vi "BMU诊断标定.vi"(8 "CAN端口":u16(ring), 9 "设备索引号":u16(ring), 10 "CAN卡类型":u32(ring)=21) -> ()   [LabVIEW 2013] (continued)
                n969 = Index Array(array=w1309, index=5 ("索引")) -> (element=w1308:bool)
                n970 = Not(x=w1317) -> (.not. x?=w1316:bool)
              }
              frame "温度起始值" {
                w1353 = 2
                w1355 = FALSE
                n971 = property on="电池实际容量(A)" class="DigNum (严格)"("Disabled"=w1353) -> ()  [unwired: 2 in, 2 out]
                n972 = property on="使用者" class="DigNum (严格)"("Disabled"=w1353) -> ()  [unwired: 2 in, 2 out]
                n973 = property on="SOH(%)" class="DigNum (严格)"("Disabled"=w1353) -> ()  [unwired: 2 in, 2 out]
                n974 = property on="电池额定容量(A)" class="DigNum (严格)"("Disabled"=w1353) -> ()  [unwired: 2 in, 2 out]
                n975 = property on="SOC(%)" class="DigNum (严格)"("Disabled"=w1353) -> ()  [unwired: 2 in, 2 out]
                n976 = local read "从板个数"() -> (w1351:dbl)
                n977 = property on="系统时钟" class="Str"("Disabled"=w1353) -> ()  [unwired: 2 in, 2 out]
                n978 = property on="配置文件版本" class="Str"("Disabled"=w1353) -> ()  [unwired: 2 in, 2 out]
                n979 = property on="车架(牌)号" class="Str"("Disabled"=w1353) -> ()  [unwired: 2 in, 2 out]
                n980 = property on="产品编号" class="Str"("Disabled"=w1353) -> ()  [unwired: 2 in, 2 out]
                n981 = control-ref of="项目信息"() -> (w1352:refnum<vi>)
                n982 = stacked-sequence {
                  tunnel: w1352 -> [w1364 w1367 w1380]
                  tunnel: w1351 -> [w1357 w1366 w1379]
                  frame #0 {
                    n983 = Multiply(x=w1357, y=3.0) -> (x*y=w1359:dbl)
                    n984 = Compound Arithmetic op=ADD(23.0 ("值"), w1359) -> (w1361:dbl)
                    n985 = Bundle(w1361, 0) -> (w1363:cluster{dbl, i32})  [unwired: 1 out]
                    n986 = property class="Tbl (严格)"(reference=w1364, "Index Values"=w1363) -> ()  [unwired: 1 in, 2 out]
                  }
                  frame #1 {
                    n987 = for {
                      N: 10 -> [_]
                      tunnel: w1367 -> [w1377]
                      tunnel: w1366 -> [w1372]
                      i -> [w1371]
                      n988 = Multiply(x=4.0, y=w1372) -> (x*y=w1369:dbl)
                      n989 = Compound Arithmetic op=ADD(24.0 ("值"), w1369, w1371) -> (w1374:dbl)
                      n990 = Bundle(w1374, 0) -> (w1376:cluster{dbl, i32})  [unwired: 1 out]
                      n991 = property class="Tbl (严格)"(reference=w1377, "Active Cell"=w1376, "Cell BG Color"=u32 16448250) -> ()  [unwired: 1 in, 2 out]
                    }
                  }
                  frame #2 {
                    n992 = Increment(x=w1379) -> (x+1=w1378:dbl)
                    n993 = for {
                      N: w1378 -> [_]
                      tunnel: w1380 -> [w1390]
                      tunnel: w1379 -> [w1385]
                      i -> [w1384]
                      n994 = Multiply(x=3.0, y=w1385) -> (x*y=w1382:dbl)
                      n995 = Compound Arithmetic op=ADD(23.0 ("值"), w1382, w1384) -> (w1387:dbl)
                      n996 = Bundle(w1387, 0) -> (w1389:cluster{dbl, i32})  [unwired: 1 out]
                      n997 = property class="Tbl (严格)"(reference=w1390, "Active Cell"=w1389, "Cell BG Color"=u32 6618880) -> ()  [unwired: 1 in, 2 out]
                    }
                  }
                }
                n998 = Select(t=0, s=w1342, f=1) -> (s? t:f=w1341:i32)
                n999 = property on="从板个数" class="DigNum (严格)"("NumText.BGColor"=u32 13816530) -> ()  [unwired: 2 in, 2 out]
                n1000 = property on="项目信息" class="Tbl (严格)"("Disabled"=w1341) -> ()  [unwired: 2 in, 2 out]
                n1001 = global read "功能码全局.vi" "主板项目信息5"() -> (w1349:bool[])
                n1002 = global read "功能码全局.vi" "主板项目信息6"() -> (w1347:bool[])
                n1003 = Index Array(array=w1349, index=5 ("索引")) -> (element=w1346:bool)
                n1004 = Index Array(array=w1347, index=6 ("索引")) -> (element=w1345:bool)
                n1005 = Not(x=w1355) -> (.not. x?=w1354:bool)
              }
              frame "保险位置" {
                w1403 = 2
                w1405 = FALSE
                n1006 = property on="电池实际容量(A)" class="DigNum (严格)"("Disabled"=w1403) -> ()  [unwired: 2 in, 2 out]
                n1007 = property on="使用者" class="DigNum (严格)"("Disabled"=w1403) -> ()  [unwired: 2 in, 2 out]
                n1008 = property on="SOH(%)" class="DigNum (严格)"("Disabled"=w1403) -> ()  [unwired: 2 in, 2 out]
                n1009 = property on="电池额定容量(A)" class="DigNum (严格)"("Disabled"=w1403) -> ()  [unwired: 2 in, 2 out]
                n1010 = property on="SOC(%)" class="DigNum (严格)"("Disabled"=w1403) -> ()  [unwired: 2 in, 2 out]
                n1011 = local read "从板个数"() -> (w1401:dbl)
                n1012 = property on="系统时钟" class="Str"("Disabled"=w1403) -> ()  [unwired: 2 in, 2 out]
                n1013 = property on="配置文件版本" class="Str"("Disabled"=w1403) -> ()  [unwired: 2 in, 2 out]
                n1014 = property on="车架(牌)号" class="Str"("Disabled"=w1403) -> ()  [unwired: 2 in, 2 out]
                n1015 = property on="产品编号" class="Str"("Disabled"=w1403) -> ()  [unwired: 2 in, 2 out]
                n1016 = control-ref of="项目信息"() -> (w1402:refnum<vi>)
                n1017 = stacked-sequence {
                  tunnel: w1402 -> [w1414 w1417]
                  tunnel: w1401 -> [w1407 w1416]
                  frame #0 {
                    n1018 = Multiply(x=w1407, y=4.0) -> (x*y=w1409:dbl)
                    n1019 = Compound Arithmetic op=ADD(24.0 ("值"), w1409) -> (w1411:dbl)
                    n1020 = Bundle(w1411, 0) -> (w1413:cluster{dbl, i32})  [unwired: 1 out]
                    n1021 = property class="Tbl (严格)"(reference=w1414, "Index Values"=w1413) -> ()  [unwired: 1 in, 2 out]
                  }
                  frame #1 {
                    n1022 = for {
                      N: 20 -> [_]
                      tunnel: w1417 -> [w1427]
                      tunnel: w1416 -> [w1422]
                      i -> [w1421]
                      n1023 = Multiply(x=4.0, y=w1422) -> (x*y=w1419:dbl)
                      n1024 = Compound Arithmetic op=ADD(24.0 ("值"), w1419, w1421) -> (w1424:dbl)
                      n1025 = Bundle(w1424, 0) -> (w1426:cluster{dbl, i32})  [unwired: 1 out]
                      n1026 = property class="Tbl (严格)"(reference=w1427, "Active Cell"=w1426, "Cell BG Color"=u32 6618880) -> ()  [unwired: 1 in, 2 out]
                    }
                  }
                }
                n1027 = property on="从板个数" class="DigNum (严格)"("NumText.BGColor"=u32 13816530) -> ()  [unwired: 2 in, 2 out]
                n1028 = Select(t=0, s=w1394, f=1) -> (s? t:f=w1392:i32)
                n1029 = global read "功能码全局.vi" "主板项目信息4"() -> (w1399:bool[])
                n1030 = property on="项目信息" class="Tbl (严格)"("Disabled"=w1392) -> ()  [unwired: 2 in, 2 out]
                n1031 = Index Array(array=w1399, index #1=5 ("索引"), index #2=6 ("索引")) -> (element #1=w1397:bool, element #2=w1396:bool)
                n1032 = Not(x=w1405) -> (.not. x?=w1404:bool)
              }
              frame "SOC" {
                w1438 = 2
                w1440 = FALSE
                n1033 = property on="电池实际容量(A)" class="DigNum (严格)"("Disabled"=w1438) -> ()  [unwired: 2 in, 2 out]
                n1034 = property on="使用者" class="DigNum (严格)"("Disabled"=w1438) -> ()  [unwired: 2 in, 2 out]
                n1035 = property on="SOH(%)" class="DigNum (严格)"("Disabled"=w1438) -> ()  [unwired: 2 in, 2 out]
                n1036 = property on="电池额定容量(A)" class="DigNum (严格)"("Disabled"=w1438) -> ()  [unwired: 2 in, 2 out]
                n1037 = property on="从板个数" class="DigNum (严格)"("NumText.BGColor"=u32 13816530) -> ()  [unwired: 2 in, 2 out]
                n1038 = property on="系统时钟" class="Str"("Disabled"=w1438) -> ()  [unwired: 2 in, 2 out]
                n1039 = property on="配置文件版本" class="Str"("Disabled"=w1438) -> ()  [unwired: 2 in, 2 out]
                n1040 = property on="车架(牌)号" class="Str"("Disabled"=w1438) -> ()  [unwired: 2 in, 2 out]
                n1041 = property on="项目信息" class="Tbl (严格)"("Disabled"=w1438) -> ()  [unwired: 2 in, 2 out]
                n1042 = property on="产品编号" class="Str"("Disabled"=w1438) -> ()  [unwired: 2 in, 2 out]
                n1043 = Select(t=0, s=w1430, f=0) -> (s? t:f=w1429:i32)
                n1044 = property on="SOC(%)" class="DigNum (严格)"("Disabled"=w1429) -> ()  [unwired: 2 in, 2 out]
                n1045 = property on="项目信息2" class="Clust (严格)"("DisabledEnum"=w1429) -> ()  [unwired: 2 in, 2 out]
                n1046 = global read "功能码全局.vi" "主板项目信息7"() -> (w1436:bool[])
                n1047 = Index Array(array=w1436, index #1=2 ("索引"), index #2=5 ("索引")) -> (element #1=w1434:bool, element #2=w1433:bool)
                n1048 = Not(x=w1440) -> (.not. x?=w1439:bool)
              }
              frame "电池额定实际容量" {
                w1452 = 2
                w1454 = FALSE
                n1049 = property on="使用者" class="DigNum (严格)"("Disabled"=w1452) -> ()  [unwired: 2 in, 2 out]
                n1050 = property on="SOH(%)" class="DigNum (严格)"("Disabled"=w1452) -> ()  [unwired: 2 in, 2 out]
                n1051 = property on="SOC(%)" class="DigNum (严格)"("Disabled"=w1452) -> ()  [unwired: 2 in, 2 out]
                n1052 = property on="从板个数" class="DigNum (严格)"("NumText.BGColor"=u32 13816530) -> ()  [unwired: 2 in, 2 out]
                n1053 = property on="系统时钟" class="Str"("Disabled"=w1452) -> ()  [unwired: 2 in, 2 out]
                n1054 = property on="配置文件版本" class="Str"("Disabled"=w1452) -> ()  [unwired: 2 in, 2 out]
                n1055 = property on="车架(牌)号" class="Str"("Disabled"=w1452) -> ()  [unwired: 2 in, 2 out]
                n1056 = property on="项目信息" class="Tbl (严格)"("Disabled"=w1452) -> ()  [unwired: 2 in, 2 out]
                n1057 = property on="产品编号" class="Str"("Disabled"=w1452) -> ()  [unwired: 2 in, 2 out]
                n1058 = Select(t=0, s=w1444, f=1) -> (s? t:f=w1443:i32)
                n1059 = property on="电池实际容量(A)" class="DigNum (严格)"("Disabled"=w1443) -> ()  [unwired: 2 in, 2 out]
                n1060 = property on="电池额定容量(A)" class="DigNum (严格)"("Disabled"=w1443) -> ()  [unwired: 2 in, 2 out]
                n1061 = property on="项目信息2" class="Clust (严格)"("DisabledEnum"=w1443) -> ()  [unwired: 2 in, 2 out]
                n1062 = global read "功能码全局.vi" "主板项目信息7"() -> (w1450:bool[])
                n1063 = Index Array(array=w1450, index #1=3 ("索引"), index #2=6 ("索引")) -> (element #1=w1448:bool, element #2=w1447:bool)
                n1064 = Not(x=w1454) -> (.not. x?=w1453:bool)
              }
              frame "配置文件版本" {
                w1467 = 2
                w1469 = FALSE
                n1065 = property on="使用者" class="DigNum (严格)"("Disabled"=w1467) -> ()  [unwired: 2 in, 2 out]
                n1066 = property on="SOH(%)" class="DigNum (严格)"("Disabled"=w1467) -> ()  [unwired: 2 in, 2 out]
                n1067 = property on="SOC(%)" class="DigNum (严格)"("Disabled"=w1467) -> ()  [unwired: 2 in, 2 out]
                n1068 = property on="电池实际容量(A)" class="DigNum (严格)"("Disabled"=w1467) -> ()  [unwired: 2 in, 2 out]
                n1069 = property on="从板个数" class="DigNum (严格)"("NumText.BGColor"=u32 13816530) -> ()  [unwired: 2 in, 2 out]
                n1070 = property on="电池额定容量(A)" class="DigNum (严格)"("Disabled"=w1467) -> ()  [unwired: 2 in, 2 out]
                n1071 = property on="系统时钟" class="Str"("Disabled"=w1467) -> ()  [unwired: 2 in, 2 out]
                n1072 = property on="车架(牌)号" class="Str"("Disabled"=w1467) -> ()  [unwired: 2 in, 2 out]
                n1073 = property on="项目信息" class="Tbl (严格)"("Disabled"=w1467) -> ()  [unwired: 2 in, 2 out]
                n1074 = property on="产品编号" class="Str"("Disabled"=w1467) -> ()  [unwired: 2 in, 2 out]
                n1075 = Select(t=0, s=w1458, f=1) -> (s? t:f=w1457:i32)
                n1076 = property on="项目信息2" class="Clust (严格)"("DisabledEnum"=w1457) -> ()  [unwired: 2 in, 2 out]
                n1077 = property on="配置文件版本" class="Str"("Disabled"=w1457) -> ()  [unwired: 2 in, 2 out]
                n1078 = global read "功能码全局.vi" "主板项目信息5"() -> (w1465:bool[])
                n1079 = global read "功能码全局.vi" "主板项目信息6"() -> (w1464:bool[])
                n1080 = Index Array(array=w1465, index=6 ("索引")) -> (element=w1462:bool)
                n1081 = Index Array(array=w1464, index=7 ("索引")) -> (element=w1461:bool)
                n1082 = Not(x=w1469) -> (.not. x?=w1468:bool)
              }
              frame "参数修改记录" {
                w1482 = 2
                w1484 = FALSE
                n1083 = property on="SOH(%)" class="DigNum (严格)"("Disabled"=w1482) -> ()  [unwired: 2 in, 2 out]
                n1084 = property on="SOC(%)" class="DigNum (严格)"("Disabled"=w1482) -> ()  [unwired: 2 in, 2 out]
                n1085 = property on="电池实际容量(A)" class="DigNum (严格)"("Disabled"=w1482) -> ()  [unwired: 2 in, 2 out]
                n1086 = property on="电池额定容量(A)" class="DigNum (严格)"("Disabled"=w1482) -> ()  [unwired: 2 in, 2 out]
                n1087 = property on="从板个数" class="DigNum (严格)"("NumText.BGColor"=u32 13816530) -> ()  [unwired: 2 in, 2 out]
                n1088 = property on="系统时钟" class="Str"("Disabled"=w1482) -> ()  [unwired: 2 in, 2 out]
                n1089 = property on="车架(牌)号" class="Str"("Disabled"=w1482) -> ()  [unwired: 2 in, 2 out]
                n1090 = property on="配置文件版本" class="Str"("Disabled"=w1482) -> ()  [unwired: 2 in, 2 out]
                n1091 = property on="项目信息" class="Tbl (严格)"("Disabled"=w1482) -> ()  [unwired: 2 in, 2 out]
                n1092 = property on="产品编号" class="Str"("Disabled"=w1482) -> ()  [unwired: 2 in, 2 out]
                n1093 = Select(t=0, s=w1473, f=1) -> (s? t:f=w1472:i32)
                n1094 = property on="使用者" class="DigNum (严格)"("Disabled"=w1472) -> ()  [unwired: 2 in, 2 out]
                n1095 = property on="项目信息2" class="Clust (严格)"("DisabledEnum"=w1472) -> ()  [unwired: 2 in, 2 out]
                n1096 = global read "功能码全局.vi" "主板项目信息7"() -> (w1479:bool[])
                n1097 = global read "功能码全局.vi" "主板项目信息5"() -> (w1480:bool[])
                n1098 = Index Array(array=w1479, index=0 ("索引")) -> (element=w1477:bool)
                n1099 = Index Array(array=w1480, index=7 ("索引")) -> (element=w1476:bool)
                n1100 = Not(x=w1484) -> (.not. x?=w1483:bool)
              }
              frame "车牌号" {
                w1497 = 2
                w1499 = FALSE
                n1101 = property on="SOH(%)" class="DigNum (严格)"("Disabled"=w1497) -> ()  [unwired: 2 in, 2 out]
                n1102 = property on="使用者" class="DigNum (严格)"("Disabled"=w1497) -> ()  [unwired: 2 in, 2 out]
                n1103 = property on="SOC(%)" class="DigNum (严格)"("Disabled"=w1497) -> ()  [unwired: 2 in, 2 out]
                n1104 = property on="电池实际容量(A)" class="DigNum (严格)"("Disabled"=w1497) -> ()  [unwired: 2 in, 2 out]
                n1105 = property on="电池额定容量(A)" class="DigNum (严格)"("Disabled"=w1497) -> ()  [unwired: 2 in, 2 out]
                n1106 = property on="从板个数" class="DigNum (严格)"("NumText.BGColor"=u32 13816530) -> ()  [unwired: 2 in, 2 out]
                n1107 = property on="系统时钟" class="Str"("Disabled"=w1497) -> ()  [unwired: 2 in, 2 out]
                n1108 = property on="配置文件版本" class="Str"("Disabled"=w1497) -> ()  [unwired: 2 in, 2 out]
                n1109 = property on="项目信息" class="Tbl (严格)"("Disabled"=w1497) -> ()  [unwired: 2 in, 2 out]
                n1110 = property on="产品编号" class="Str"("Disabled"=w1497) -> ()  [unwired: 2 in, 2 out]
                n1111 = Select(t=0, s=w1488, f=1) -> (s? t:f=w1487:i32)
                n1112 = property on="车架(牌)号" class="Str"("Disabled"=w1487) -> ()  [unwired: 2 in, 2 out]
                n1113 = property on="项目信息2" class="Clust (严格)"("DisabledEnum"=w1487) -> ()  [unwired: 2 in, 2 out]
                n1114 = global read "功能码全局.vi" "主板项目信息7"() -> (w1494:bool[])
                n1115 = global read "功能码全局.vi" "主板项目信息6"() -> (w1495:bool[])
                n1116 = Index Array(array=w1494, index=1 ("索引")) -> (element=w1492:bool)
                n1117 = Index Array(array=w1495, index=0 ("索引")) -> (element=w1491:bool)
                n1118 = Not(x=w1499) -> (.not. x?=w1498:bool)
              }
              frame "SOH" {
                w1511 = 2
                w1513 = FALSE
                n1119 = property on="使用者" class="DigNum (严格)"("Disabled"=w1511) -> ()  [unwired: 2 in, 2 out]
                n1120 = property on="SOC(%)" class="DigNum (严格)"("Disabled"=w1511) -> ()  [unwired: 2 in, 2 out]
                n1121 = property on="电池实际容量(A)" class="DigNum (严格)"("Disabled"=w1511) -> ()  [unwired: 2 in, 2 out]
                n1122 = property on="电池额定容量(A)" class="DigNum (严格)"("Disabled"=w1511) -> ()  [unwired: 2 in, 2 out]
                n1123 = property on="从板个数" class="DigNum (严格)"("NumText.BGColor"=u32 13816530) -> ()  [unwired: 2 in, 2 out]
                n1124 = property on="系统时钟" class="Str"("Disabled"=w1511) -> ()  [unwired: 2 in, 2 out]
                n1125 = property on="配置文件版本" class="Str"("Disabled"=w1511) -> ()  [unwired: 2 in, 2 out]
                n1126 = property on="项目信息" class="Tbl (严格)"("Disabled"=w1511) -> ()  [unwired: 2 in, 2 out]
                n1127 = property on="产品编号" class="Str"("Disabled"=w1511) -> ()  [unwired: 2 in, 2 out]
                n1128 = property on="车架(牌)号" class="Str"("Disabled"=w1511) -> ()  [unwired: 2 in, 2 out]
                n1129 = Select(t=0, s=w1503, f=1) -> (s? t:f=w1502:i32)
                n1130 = property on="项目信息2" class="Clust (严格)"("DisabledEnum"=w1502) -> ()  [unwired: 2 in, 2 out]
                n1131 = property on="SOH(%)" class="DigNum (严格)"("Disabled"=w1502) -> ()  [unwired: 2 in, 2 out]
                n1132 = global read "功能码全局.vi" "主板项目信息7"() -> (w1510:bool[])
                n1133 = Index Array(array=w1510, index #1=4 ("索引"), index #2=7 ("索引")) -> (element #1=w1507:bool, element #2=w1506:bool)
                n1134 = Not(x=w1513) -> (.not. x?=w1512:bool)
              }
              frame "SOC过低(2)", "SOC过高(2)", "SOH过低(2)", "充电电流过高(2)", "单体电压过低(2)", "单体电压过高(2)", "单组电压不均衡(2)", "单组温度不均衡(2)", "二级故障阀值", "放电电流过高(2)", "极柱温度过高(2)", "内阻过大(2)", "温度过低(2)", "温度过高(2)", "整组电压不均衡(2)", "整组温度不均衡(2)", "总电压过低(2)", "总电压过高(2)" {
                w1525 = FALSE
                n1135 = property on="从板个数" class="DigNum (严格)"("NumText.BGColor"=u32 13816530) -> ()  [unwired: 2 in, 2 out]
                n1136 = Select(t=0, s=w1517, f=1) -> (s? t:f=w1516:i32)
                n1137 = property on="一级故障 2" class="Clust (严格)"("DisabledEnum"=w1516) -> ()  [unwired: 2 in, 2 out]
                n1138 = global read "功能码全局.vi" "主板故障阀值9"() -> (w1523:bool[])
                n1139 = Index Array(array=w1523, index #1=3 ("索引"), index #2=6 ("索引")) -> (element #1=w1521:bool, element #2=w1520:bool)
                n1140 = Not(x=w1525) -> (.not. x?=w1526:bool)
              }
              frame "SOC过低(3)", "SOC过高(3)", "SOH过低(3)", "充电电流过高(3)", "单体电压过低(3)", "单体电压过高(3)", "单组电压不均衡(3)", "单组温度不均衡(3)", "放电电流过高(3)", "极柱温度过高(3)", "内阻过大(3)", "三级故障阀值", "温度过低(3)", "温度过高(3)", "整组电压不均衡(3)", "整组温度不均衡(3)", "总电压过低(3)", "总电压过高(3)" {
                w1539 = FALSE
                n1141 = property on="从板个数" class="DigNum (严格)"("NumText.BGColor"=u32 13816530) -> ()  [unwired: 2 in, 2 out]
                n1142 = Select(t=0, s=w1530, f=1) -> (s? t:f=w1529:i32)
                n1143 = property on="一级故障 3" class="Clust (严格)"("DisabledEnum"=w1529) -> ()  [unwired: 2 in, 2 out]
                n1144 = global read "功能码全局.vi" "主板故障阀值9"() -> (w1536:bool[])
                n1145 = Index Array(array=w1536, index #1=4 ("索引"), index #2=7 ("索引")) -> (element #1=w1534:bool, element #2=w1533:bool)
                n1146 = Not(x=w1539) -> (.not. x?=w1538:bool)
              }
              frame "SOC过低", "SOC过高", "SOH过低", "充电电流过高", "单体电压过低", "单体电压过高", "单组电压不均衡", "单组温度不均衡", "放电电流过高", "极柱温度过高", "内阻过大", "温度过低", "温度过高", "一级故障阀值", "整组电压不均衡", "整组温度不均衡", "总电压过低", "总电压过高" {
                w1552 = FALSE
                n1147 = Select(t=0, s=w1543, f=1) -> (s? t:f=w1542:i32)
                n1148 = property on="从板个数" class="DigNum (严格)"("NumText.BGColor"=u32 13816530) -> ()  [unwired: 2 in, 2 out]
                n1149 = property on="一级故障" class="Clust (严格)"("DisabledEnum"=w1542) -> ()  [unwired: 2 in, 2 out]
                n1150 = global read "功能码全局.vi" "主板故障阀值9"() -> (w1549:bool[])
                n1151 = Index Array(array=w1549, index #1=2 ("索引"), index #2=5 ("索引")) -> (element #1=w1547:bool, element #2=w1546:bool)
                n1152 = Not(x=w1552) -> (.not. x?=w1551:bool)
              }
              frame "充电控制参数", "电流步长", "最大允许充电电流", "最大允许充电温度", "最大允许单体电压", "最大允许总电压", "最小允许充电电流", "最小允许充电温度", "最小允许单体电压" {
                w1555 = 2
                w1566 = FALSE
                n1153 = property on="从板个数" class="DigNum (严格)"("NumText.BGColor"=u32 13816530) -> ()  [unwired: 2 in, 2 out]
                n1154 = property on="风机开启温度" class="DigNum (严格)"("Disabled"=w1555) -> ()  [unwired: 2 in, 2 out]
                n1155 = property on="风机关闭温度" class="DigNum (严格)"("Disabled"=w1555) -> ()  [unwired: 2 in, 2 out]
                n1156 = property on="加热开启温度" class="DigNum (严格)"("Disabled"=w1555) -> ()  [unwired: 2 in, 2 out]
                n1157 = property on="加热关闭温度" class="DigNum (严格)"("Disabled"=w1555) -> ()  [unwired: 2 in, 2 out]
                n1158 = property on="风机开启温差" class="DigNum (严格)"("Disabled"=w1555) -> ()  [unwired: 2 in, 2 out]
                n1159 = property on="风机关闭温差" class="DigNum (严格)"("Disabled"=w1555) -> ()  [unwired: 2 in, 2 out]
                n1160 = property on="加热控制参数" class="Clust (严格)"("DisabledEnum"=w1555) -> ()  [unwired: 2 in, 2 out]
                n1161 = Select(t=0, s=w1557, f=1) -> (s? t:f=w1556:i32)
                n1162 = property on="最大允许总电压" class="DigNum (严格)"("Disabled"=w1556) -> ()  [unwired: 2 in, 2 out]
                n1163 = property on="最大允许充电温度" class="DigNum (严格)"("Disabled"=w1556) -> ()  [unwired: 2 in, 2 out]
                n1164 = property on="最小允许充电温度" class="DigNum (严格)"("Disabled"=w1556) -> ()  [unwired: 2 in, 2 out]
                n1165 = property on="电流步长" class="DigNum (严格)"("Disabled"=w1556) -> ()  [unwired: 2 in, 2 out]
                n1166 = property on="最大允许单体电压" class="DigNum (严格)"("Disabled"=w1556) -> ()  [unwired: 2 in, 2 out]
                n1167 = property on="最小允许单体电压" class="DigNum (严格)"("Disabled"=w1556) -> ()  [unwired: 2 in, 2 out]
                n1168 = property on="最大允许充电电流" class="DigNum (严格)"("Disabled"=w1556) -> ()  [unwired: 2 in, 2 out]
                n1169 = property on="最小允许充电电流" class="DigNum (严格)"("Disabled"=w1556) -> ()  [unwired: 2 in, 2 out]
                n1170 = global read "功能码全局.vi" "主板控制类信息10"() -> (w1563:bool[])
                n1171 = Index Array(array=w1563, index #1=5 ("索引"), index #2=7 ("索引")) -> (element #1=w1561:bool, element #2=w1560:bool)
                n1172 = Not(x=w1566) -> (.not. x?=w1565:bool)
              }
              frame "风机关闭温差", "风机关闭温度", "风机开启温差", "风机开启温度", "加热关闭温差", "加热关闭温度", "加热开启温度", "加热控制参数" {
                w1578 = 2
                w1580 = FALSE
                n1173 = Select(t=0, s=w1570, f=1) -> (s? t:f=w1569:i32)
                n1174 = property on="从板个数" class="DigNum (严格)"("NumText.BGColor"=u32 13816530) -> ()  [unwired: 2 in, 2 out]
                n1175 = property on="加热控制参数" class="Clust (严格)"("DisabledEnum"=w1569) -> ()  [unwired: 2 in, 2 out]
                n1176 = property on="风机开启温度" class="DigNum (严格)"("Disabled"=w1569) -> ()  [unwired: 2 in, 2 out]
                n1177 = property on="风机关闭温度" class="DigNum (严格)"("Disabled"=w1569) -> ()  [unwired: 2 in, 2 out]
                n1178 = property on="加热开启温度" class="DigNum (严格)"("Disabled"=w1569) -> ()  [unwired: 2 in, 2 out]
                n1179 = property on="加热关闭温度" class="DigNum (严格)"("Disabled"=w1569) -> ()  [unwired: 2 in, 2 out]
                n1180 = property on="风机开启温差" class="DigNum (严格)"("Disabled"=w1569) -> ()  [unwired: 2 in, 2 out]
                n1181 = property on="风机关闭温差" class="DigNum (严格)"("Disabled"=w1569) -> ()  [unwired: 2 in, 2 out]
                n1182 = property on="最大允许总电压" class="DigNum (严格)"("Disabled"=w1578) -> ()  [unwired: 2 in, 2 out]
                n1183 = property on="最大允许充电温度" class="DigNum (严格)"("Disabled"=w1578) -> ()  [unwired: 2 in, 2 out]
                n1184 = property on="最小允许充电温度" class="DigNum (严格)"("Disabled"=w1578) -> ()  [unwired: 2 in, 2 out]
                n1185 = property on="电流步长" class="DigNum (严格)"("Disabled"=w1578) -> ()  [unwired: 2 in, 2 out]
                n1186 = property on="最大允许单体电压" class="DigNum (严格)"("Disabled"=w1578) -> ()  [unwired: 2 in, 2 out]
                n1187 = property on="最小允许单体电压" class="DigNum (严格)"("Disabled"=w1578) -> ()  [unwired: 2 in, 2 out]
                n1188 = property on="最大允许充电电流" class="DigNum (严格)"("Disabled"=w1578) -> ()  [unwired: 2 in, 2 out]
                n1189 = property on="最小允许充电电流" class="DigNum (严格)"("Disabled"=w1578) -> ()  [unwired: 2 in, 2 out]
                n1190 = global read "功能码全局.vi" "主板控制类信息10"() -> (w1576:bool[])
                n1191 = Index Array(array=w1576, index #1=4 ("索引"), index #2=6 ("索引")) -> (element #1=w1574:bool, element #2=w1573:bool)
                n1192 = Not(x=w1580) -> (.not. x?=w1579:bool)
              }
              frame "电池信息" {
                w1593 = FALSE
                n1193 = Select(t=0, s=w1584, f=1) -> (s? t:f=w1583:i32)
                n1194 = property on="电池串联" class="DigNum (严格)"("Disabled"=w1583) -> ()  [unwired: 2 in, 2 out]
                n1195 = property on="电池并联" class="DigNum (严格)"("Disabled"=w1583) -> ()  [unwired: 2 in, 2 out]
                n1196 = property on="电池包额定容量" class="DigNum (严格)"("Disabled"=w1583) -> ()  [unwired: 2 in, 2 out]
                n1197 = property on="电池包额定能量(kWh)" class="DigNum (严格)"("Disabled"=w1583) -> ()  [unwired: 2 in, 2 out]
                n1198 = property on="电池包额定总电压" class="DigNum (严格)"("Disabled"=w1583) -> ()  [unwired: 2 in, 2 out]
                n1199 = property on="实际容量" class="DigNum (严格)"("Disabled"=w1583) -> ()  [unwired: 2 in, 2 out]
                n1200 = property on="电池包组号" class="Str"("Disabled"=w1583) -> ()  [unwired: 2 in, 2 out]
                n1201 = property on="电池生产日期" class="Str"("Disabled"=w1583) -> ()  [unwired: 2 in, 2 out]
                n1202 = property on="电池厂家" class="Str"("Disabled"=w1583) -> ()  [unwired: 2 in, 2 out]
                n1203 = property on="电池类型" class="Str"("Disabled"=w1583) -> ()  [unwired: 2 in, 2 out]
                n1204 = property on="累计充电总安时" class="DigNum (严格)"("Disabled"=w1583) -> ()  [unwired: 2 in, 2 out]
                n1205 = property on="累计放电总安时" class="DigNum (严格)"("Disabled"=w1583) -> ()  [unwired: 2 in, 2 out]
                n1206 = property on="电池放空次数" class="DigNum (严格)"("Disabled"=w1583) -> ()  [unwired: 2 in, 2 out]
                n1207 = property on="电池充满次数" class="DigNum (严格)"("Disabled"=w1583) -> ()  [unwired: 2 in, 2 out]
                n1208 = property on="电池充电次数" class="DigNum (严格)"("Disabled"=w1583) -> ()  [unwired: 2 in, 2 out]
                n1209 = property on="电池信息" class="Clust (严格)"("DisabledEnum"=w1583) -> ()  [unwired: 2 in, 2 out]
                n1210 = global read "功能码全局.vi" "主板版本号11"() -> (w1590:bool[])
                n1211 = property on="从板个数" class="DigNum (严格)"("NumText.BGColor"=u32 13816530) -> ()  [unwired: 2 in, 2 out]
                n1212 = Index Array(array=w1590, index #1=0 ("索引"), index #2=1 ("索引")) -> (element #1=w1588:bool, element #2=w1587:bool)
                n1213 = Not(x=w1593) -> (.not. x?=w1592:bool)
              }
              frame "电池信息1" {
                w1605 = 2
                w1607 = FALSE
                n1214 = Select(t=0, s=w1597, f=1) -> (s? t:f=w1596:i32)
                n1215 = property on="电池信息" class="Clust (严格)"("DisabledEnum"=w1596) -> ()  [unwired: 2 in, 2 out]
                n1216 = property on="电池生产日期" class="Str"("Disabled"=w1596) -> ()  [unwired: 2 in, 2 out]
                n1217 = property on="电池厂家" class="Str"("Disabled"=w1596) -> ()  [unwired: 2 in, 2 out]
                n1218 = property on="电池类型" class="Str"("Disabled"=w1596) -> ()  [unwired: 2 in, 2 out]
                n1219 = property on="电池串联" class="DigNum (严格)"("Disabled"=w1596) -> ()  [unwired: 2 in, 2 out]
                n1220 = property on="电池并联" class="DigNum (严格)"("Disabled"=w1596) -> ()  [unwired: 2 in, 2 out]
                n1221 = property on="电池包额定容量" class="DigNum (严格)"("Disabled"=w1596) -> ()  [unwired: 2 in, 2 out]
                n1222 = property on="电池包额定能量(kWh)" class="DigNum (严格)"("Disabled"=w1596) -> ()  [unwired: 2 in, 2 out]
                n1223 = property on="电池包额定总电压" class="DigNum (严格)"("Disabled"=w1596) -> ()  [unwired: 2 in, 2 out]
                n1224 = property on="实际容量" class="DigNum (严格)"("Disabled"=w1596) -> ()  [unwired: 2 in, 2 out]
                n1225 = property on="累计充电总安时" class="DigNum (严格)"("Disabled"=w1605) -> ()  [unwired: 2 in, 2 out]
                n1226 = property on="累计放电总安时" class="DigNum (严格)"("Disabled"=w1605) -> ()  [unwired: 2 in, 2 out]
                n1227 = property on="电池放空次数" class="DigNum (严格)"("Disabled"=w1605) -> ()  [unwired: 2 in, 2 out]
                n1228 = property on="电池充满次数" class="DigNum (严格)"("Disabled"=w1605) -> ()  [unwired: 2 in, 2 out]
                n1229 = property on="电池充电次数" class="DigNum (严格)"("Disabled"=w1605) -> ()  [unwired: 2 in, 2 out]
                n1230 = property on="从板个数" class="DigNum (严格)"("NumText.BGColor"=u32 13816530) -> ()  [unwired: 2 in, 2 out]
                n1231 = property on="电池包组号" class="Str"("Disabled"=w1605) -> ()  [unwired: 2 in, 2 out]
                n1232 = global read "功能码全局.vi" "主板版本号11"() -> (w1603:bool[])
                n1233 = Index Array(array=w1603, index #1=0 ("索引"), index #2=1 ("索引")) -> (element #1=w1601:bool, element #2=w1600:bool)
                n1234 = Not(x=w1607) -> (.not. x?=w1606:bool)
              }
              frame "电池包组号" {
                w1619 = 2
                w1621 = FALSE
                n1235 = property on="电池生产日期" class="Str"("Disabled"=w1619) -> ()  [unwired: 2 in, 2 out]
                n1236 = property on="电池厂家" class="Str"("Disabled"=w1619) -> ()  [unwired: 2 in, 2 out]
                n1237 = property on="电池类型" class="Str"("Disabled"=w1619) -> ()  [unwired: 2 in, 2 out]
                n1238 = property on="电池串联" class="DigNum (严格)"("Disabled"=w1619) -> ()  [unwired: 2 in, 2 out]
                n1239 = property on="电池并联" class="DigNum (严格)"("Disabled"=w1619) -> ()  [unwired: 2 in, 2 out]
                n1240 = property on="电池包额定容量" class="DigNum (严格)"("Disabled"=w1619) -> ()  [unwired: 2 in, 2 out]
                n1241 = property on="电池包额定能量(kWh)" class="DigNum (严格)"("Disabled"=w1619) -> ()  [unwired: 2 in, 2 out]
                n1242 = property on="电池包额定总电压" class="DigNum (严格)"("Disabled"=w1619) -> ()  [unwired: 2 in, 2 out]
                n1243 = property on="实际容量" class="DigNum (严格)"("Disabled"=w1619) -> ()  [unwired: 2 in, 2 out]
                n1244 = property on="从板个数" class="DigNum (严格)"("NumText.BGColor"=u32 13816530) -> ()  [unwired: 2 in, 2 out]
                n1245 = property on="累计充电总安时" class="DigNum (严格)"("Disabled"=w1619) -> ()  [unwired: 2 in, 2 out]
                n1246 = property on="累计放电总安时" class="DigNum (严格)"("Disabled"=w1619) -> ()  [unwired: 2 in, 2 out]
                n1247 = property on="电池放空次数" class="DigNum (严格)"("Disabled"=w1619) -> ()  [unwired: 2 in, 2 out]
                n1248 = property on="电池充满次数" class="DigNum (严格)"("Disabled"=w1619) -> ()  [unwired: 2 in, 2 out]
                n1249 = property on="电池充电次数" class="DigNum (严格)"("Disabled"=w1619) -> ()  [unwired: 2 in, 2 out]
                n1250 = Select(t=0, s=w1611, f=1) -> (s? t:f=w1610:i32)
                n1251 = property on="电池包组号" class="Str"("Disabled"=w1610) -> ()  [unwired: 2 in, 2 out]
                n1252 = property on="电池信息" class="Clust (严格)"("DisabledEnum"=w1610) -> ()  [unwired: 2 in, 2 out]
                n1253 = global read "功能码全局.vi" "主板版本号11"() -> (w1617:bool[])
                n1254 = Index Array(array=w1617, index #1=0 ("索引"), index #2=1 ("索引")) -> (element #1=w1615:bool, element #2=w1614:bool)
                n1255 = Not(x=w1621) -> (.not. x?=w1620:bool)
              }
              frame "充放电安时" {
                w1633 = 2
                w1635 = FALSE
                n1256 = property on="电池生产日期" class="Str"("Disabled"=w1633) -> ()  [unwired: 2 in, 2 out]
                n1257 = property on="电池厂家" class="Str"("Disabled"=w1633) -> ()  [unwired: 2 in, 2 out]
                n1258 = property on="电池类型" class="Str"("Disabled"=w1633) -> ()  [unwired: 2 in, 2 out]
                n1259 = property on="电池串联" class="DigNum (严格)"("Disabled"=w1633) -> ()  [unwired: 2 in, 2 out]
                n1260 = property on="电池并联" class="DigNum (严格)"("Disabled"=w1633) -> ()  [unwired: 2 in, 2 out]
                n1261 = property on="电池包额定容量" class="DigNum (严格)"("Disabled"=w1633) -> ()  [unwired: 2 in, 2 out]
                n1262 = property on="电池包额定能量(kWh)" class="DigNum (严格)"("Disabled"=w1633) -> ()  [unwired: 2 in, 2 out]
                n1263 = property on="电池包额定总电压" class="DigNum (严格)"("Disabled"=w1633) -> ()  [unwired: 2 in, 2 out]
                n1264 = property on="实际容量" class="DigNum (严格)"("Disabled"=w1633) -> ()  [unwired: 2 in, 2 out]
                n1265 = property on="从板个数" class="DigNum (严格)"("NumText.BGColor"=u32 13816530) -> ()  [unwired: 2 in, 2 out]
                n1266 = Select(t=0, s=w1625, f=1) -> (s? t:f=w1624:i32)
                n1267 = property on="电池放空次数" class="DigNum (严格)"("Disabled"=w1633) -> ()  [unwired: 2 in, 2 out]
                n1268 = property on="电池充满次数" class="DigNum (严格)"("Disabled"=w1633) -> ()  [unwired: 2 in, 2 out]
                n1269 = property on="电池充电次数" class="DigNum (严格)"("Disabled"=w1633) -> ()  [unwired: 2 in, 2 out]
                n1270 = property on="电池包组号" class="Str"("Disabled"=w1633) -> ()  [unwired: 2 in, 2 out]
                n1271 = property on="累计充电总安时" class="DigNum (严格)"("Disabled"=w1624) -> ()  [unwired: 2 in, 2 out]
                n1272 = property on="累计放电总安时" class="DigNum (严格)"("Disabled"=w1624) -> ()  [unwired: 2 in, 2 out]
                n1273 = property on="电池信息" class="Clust (严格)"("DisabledEnum"=w1624) -> ()  [unwired: 2 in, 2 out]
                n1274 = global read "功能码全局.vi" "主板版本号11"() -> (w1631:bool[])
                n1275 = Index Array(array=w1631, index #1=0 ("索引"), index #2=1 ("索引")) -> (element #1=w1629:bool, element #2=w1628:bool)
                n1276 = Not(x=w1635) -> (.not. x?=w1634:bool)
              }
              frame "电池充放电次数" {
                w1647 = 2
                w1649 = FALSE
                n1277 = property on="从板个数" class="DigNum (严格)"("NumText.BGColor"=u32 13816530) -> ()  [unwired: 2 in, 2 out]
                n1278 = property on="电池生产日期" class="Str"("Disabled"=w1647) -> ()  [unwired: 2 in, 2 out]
                n1279 = property on="电池厂家" class="Str"("Disabled"=w1647) -> ()  [unwired: 2 in, 2 out]
                n1280 = property on="电池类型" class="Str"("Disabled"=w1647) -> ()  [unwired: 2 in, 2 out]
                n1281 = property on="电池串联" class="DigNum (严格)"("Disabled"=w1647) -> ()  [unwired: 2 in, 2 out]
                n1282 = property on="电池并联" class="DigNum (严格)"("Disabled"=w1647) -> ()  [unwired: 2 in, 2 out]
                n1283 = property on="电池包额定容量" class="DigNum (严格)"("Disabled"=w1647) -> ()  [unwired: 2 in, 2 out]
                n1284 = property on="电池包额定能量(kWh)" class="DigNum (严格)"("Disabled"=w1647) -> ()  [unwired: 2 in, 2 out]
                n1285 = property on="电池包额定总电压" class="DigNum (严格)"("Disabled"=w1647) -> ()  [unwired: 2 in, 2 out]
                n1286 = property on="实际容量" class="DigNum (严格)"("Disabled"=w1647) -> ()  [unwired: 2 in, 2 out]
                n1287 = Select(t=0, s=w1639, f=1) -> (s? t:f=w1638:i32)
                n1288 = property on="电池放空次数" class="DigNum (严格)"("Disabled"=w1638) -> ()  [unwired: 2 in, 2 out]
                n1289 = property on="电池充满次数" class="DigNum (严格)"("Disabled"=w1638) -> ()  [unwired: 2 in, 2 out]
                n1290 = property on="电池充电次数" class="DigNum (严格)"("Disabled"=w1638) -> ()  [unwired: 2 in, 2 out]
                n1291 = property on="累计充电总安时" class="DigNum (严格)"("Disabled"=w1647) -> ()  [unwired: 2 in, 2 out]
                n1292 = property on="累计放电总安时" class="DigNum (严格)"("Disabled"=w1647) -> ()  [unwired: 2 in, 2 out]
                n1293 = property on="电池信息" class="Clust (严格)"("DisabledEnum"=w1638) -> ()  [unwired: 2 in, 2 out]
                n1294 = property on="电池包组号" class="Str"("Disabled"=w1647) -> ()  [unwired: 2 in, 2 out]
                n1295 = global read "功能码全局.vi" "主板版本号11"() -> (w1645:bool[])
                n1296 = Index Array(array=w1645, index #1=0 ("索引"), index #2=1 ("索引")) -> (element #1=w1643:bool, element #2=w1642:bool)
                n1297 = Not(x=w1649) -> (.not. x?=w1648:bool)
              }
              frame "假", Default {
                w1654 = FALSE
                n1298 = Not(x=w1654) -> (.not. x?=w1653:bool)
              }
            }
            n1299 = property on="单个读取" class="Bool (严格)"("Visible"=w1137) -> ()  [unwired: 2 in, 2 out]
            n1300 = property on="单个写入" class="Bool (严格)"("Visible"=w1136) -> ()  [unwired: 2 in, 2 out]
            n1301 = local write "1"(w1144) -> ()
            n1302 = local write "1 2"(w1143) -> ()
            n1303 = local write "1 3"(w1142) -> ()
            n1304 = local write "1 4"(w1141) -> ()
            n1305 = local write "1 5"(w1140) -> ()
            n1306 = local write "1 11"(w1139) -> ()
            n1307 = local write "主板2"(w1145) -> ()
          }
          event "从板选项": Mouse Down {
            n1308 = event-data() -> ("CtlRef"=w1669:refnum<vi>)  [unwired: 8 out]
            n1309 = property class="Tree (严格)"(reference=w1669) -> ("Value"=w1668:string)  [unwired: 1 in, 2 out]
            n1310 = global read "功能码全局.vi" "主板监控2"() -> (w1659:bool[])
            n1311 = Index Array(array=w1659, index=6 ("索引")) -> (element=w1657:bool)
            n1312 = case shown="\"温度个数\"" w1668 {
              tunnel: [T21."从板信息" ("等级 2") T21."从板信息" ("等级 2") T21."从板信息" ("等级 2") T21."从板信息" ("等级 2") T21."从板信息" ("等级 2") T21."从板信息" ("等级 2") T21."从板信息" ("等级 2") T21."一级故障阀值" ("等级 2") T21."二级故障阀值" ("等级 2") T21."三级故障阀值" ("等级 2") T21."快换参数" ("等级 2") T21."快换参数" ("等级 2") T21."快换参数" ("等级 2") T21."快换参数" ("等级 2") T21."快换参数" ("等级 2") T21."快换参数" ("等级 2") T21."快换参数" ("等级 2") T21."快换参数" ("等级 2") T14."均衡参数" ("等级 2") T14."均衡参数" ("等级 2") T14."均衡参数" ("等级 2") T21."从板信息" ("等级 2")] -> w1667
              tunnel: [w1680 w1690 w1704 w1719 w1754 w1791 w1828 w1852 w1865 w1878 w1891 w1917 w1931 w1947 w1964 w1981 w1999 w2018 w2035 w2048 w2062 w2077] -> w1666
              tunnel: [w1672 w1682 w1692 w1706 w1741 w1778 w1815 w1863 w1865 w1878 w1891 w1917 w1931 w1947 w1964 w1981 w1999 w2018 w2035 w2048 w2062 w2076] -> w1665
              tunnel: [w1672 w1682 w1692 w1706 w1741 w1778 w1815 w1852 w1876 w1878 w1891 w1917 w1931 w1947 w1964 w1981 w1999 w2018 w2035 w2048 w2062 w2076] -> w1664
              tunnel: [w1672 w1682 w1692 w1706 w1741 w1778 w1815 w1852 w1865 w1889 w1891 w1917 w1931 w1947 w1964 w1981 w1999 w2018 w2035 w2048 w2062 w2076] -> w1663
              tunnel: [w1672 w1682 w1692 w1706 w1741 w1778 w1815 w1852 w1865 w1878 w1915 w1929 w1945 w1962 w1979 w1997 w2016 w2033 w2035 w2048 w2062 w2076] -> w1662
              tunnel: [w1677 w1683 w1699 w1713 w1748 w1785 w1822 w1859 w1872 w1885 w1900 w1922 w1937 w1951 w1969 w1984 w2004 w2022 w2038 w2052 w2067 w2076] -> w1661
              tunnel: [w1674 w1683 w1698 w1712 w1747 w1784 w1821 w1858 w1871 w1884 w1892 w1921 w1936 w1950 w1970 w1985 w2003 w2021 w2037 w2051 w2066 w2076] -> w1660
              tunnel: w1657 -> [_ w1687 w1695 w1709 w1744 w1781 w1818 w1854 w1868 w1881 w1912 w1925 w1940 w1955 w1973 w1989 w2007 w2026 w2041 w2055 w2069 _]
              tunnel: [w1672 w1682 w1692 w1706 w1741 w1778 w1815 w1852 w1865 w1878 w1891 w1917 w1931 w1947 w1964 w1981 w1999 w2018 w2036 w2049 w2063 w2076] -> w1656
              frame "从板号" {
                w1679 = 2
                w1672 = FALSE ("1 6")
                n1313 = property on="项目信息 2" class="Tbl (严格)"("Disabled"=w1679) -> ()  [unwired: 2 in, 2 out]
                n1314 = property on="加热控制参数" class="Clust (严格)"("Disabled"=w1679) -> ()  [unwired: 2 in, 2 out]
                n1315 = property on="从板号" class="DigNum (严格)"("NumText.BGColor"=u32 6618880) -> ()  [unwired: 2 in, 2 out]
                n1316 = global read "功能码全局.vi" "16"() -> (w1676:bool[])
                n1317 = Index Array(array=w1676, index #1=4 ("索引"), index #2=6 ("索引")) -> (element #1=w1677:bool, element #2=w1674:bool)
                n1318 = Not(x=w1672) -> (.not. x?=w1680:bool)
              }
              frame "从板信息" {
                w1682 = FALSE ("1 6")
                n1319 = Select(t=0, s=w1687, f=1) -> (s? t:f=w1686:i32)
                n1320 = property on="从板号" class="DigNum (严格)"("NumText.BGColor"=u32 16777215) -> ()  [unwired: 2 in, 2 out]
                n1321 = property on="项目信息 2" class="Tbl (严格)"("Disabled"=w1686) -> ()  [unwired: 2 in, 2 out]
                n1322 = property on="加热控制参数" class="Clust (严格)"("Disabled"=w1686) -> ()  [unwired: 2 in, 2 out]
                n1323 = Not(x=w1682) -> (.not. x?=w1690:bool)
                n1324 = local read "从板项目信息"() -> (w1684:bool)
                n1325 = Not(x=w1684) -> (.not. x?=w1683:bool)
              }
              frame "风机关闭温差", "风机关闭温度", "风机开启温差", "风机开启温度", "加热关闭温差", "加热关闭温度", "加热开启温度", "加热控制参数" {
                w1692 = FALSE ("1 6")
                n1326 = property on="从板号" class="DigNum (严格)"("NumText.BGColor"=u32 16777215) -> ()  [unwired: 2 in, 2 out]
                n1327 = Select(t=0, s=w1695, f=1) -> (s? t:f=w1694:i32)
                n1328 = property on="项目信息 2" class="Tbl (严格)"("Disabled"=2) -> ()  [unwired: 2 in, 2 out]
                n1329 = property on="加热控制参数" class="Clust (严格)"("Disabled"=w1694) -> ()  [unwired: 2 in, 2 out]
                n1330 = global read "功能码全局.vi" "16"() -> (w1701:bool[])
                n1331 = Index Array(array=w1701, index #1=5 ("索引"), index #2=7 ("索引")) -> (element #1=w1699:bool, element #2=w1698:bool)
                n1332 = Not(x=w1692) -> (.not. x?=w1704:bool)
              }
              frame "电压个数" {
                w1706 = FALSE ("1 6")
                n1333 = property on="从板号" class="DigNum (严格)"("NumText.BGColor"=u32 16777215) -> ()  [unwired: 2 in, 2 out]
                n1334 = control-ref of="项目信息 2"() -> (w1717:refnum<vi>)
                n1335 = stacked-sequence {
                  tunnel: w1717 -> [w1724 w1726 w1735]
                  frame #0 {
                    n1336 = Bundle(0, 0) -> (w1723:cluster{i32, i32})  [unwired: 1 out]
                    n1337 = property class="Tbl (严格)"(reference=w1724, "Index Values"=w1723) -> ()  [unwired: 1 in, 2 out]
                  }
                  frame #1 {
                    n1338 = for {
                      N: 40 -> [_]
                      tunnel: w1726 -> [w1733]
                      i -> [w1728]
                      n1339 = Compound Arithmetic op=ADD(0 ("值"), w1728) -> (w1730:i32)
                      n1340 = Bundle(w1730, 0) -> (w1732:cluster{i32, i32})  [unwired: 1 out]
                      n1341 = property class="Tbl (严格)"(reference=w1733, "Active Cell"=w1732, "Cell BG Color"=u32 16448250) -> ()  [unwired: 1 in, 2 out]
                    }
                  }
                  frame #2 {
                    n1342 = for {
                      N: 1 -> [_]
                      tunnel: w1735 -> [w1740]
                      i -> [w1736]
                      n1343 = Bundle(w1736, 0) -> (w1739:cluster{i32, i32})  [unwired: 1 out]
                      n1344 = property class="Tbl (严格)"(reference=w1740, "Active Cell"=w1739, "Cell BG Color"=u32 6618880) -> ()  [unwired: 1 in, 2 out]
                    }
                  }
                }
                n1345 = Select(t=0, s=w1709, f=1) -> (s? t:f=w1708:i32)
                n1346 = property on="项目信息 2" class="Tbl (严格)"("Disabled"=w1708) -> ()  [unwired: 2 in, 2 out]
                n1347 = property on="加热控制参数" class="Clust (严格)"("Disabled"=2) -> ()  [unwired: 2 in, 2 out]
                n1348 = global read "功能码全局.vi" "15"() -> (w1715:bool[])
                n1349 = Index Array(array=w1715, index #1=0 ("索引"), index #2=4 ("索引")) -> (element #1=w1713:bool, element #2=w1712:bool)
                n1350 = Not(x=w1706) -> (.not. x?=w1719:bool)
              }
              frame "通道电压节数" {
                w1741 = FALSE ("1 6")
                n1351 = property on="从板号" class="DigNum (严格)"("NumText.BGColor"=u32 16777215) -> ()  [unwired: 2 in, 2 out]
                n1352 = control-ref of="项目信息 2"() -> (w1752:refnum<vi>)
                n1353 = stacked-sequence {
                  tunnel: w1752 -> [w1759 w1761 w1770]
                  frame #0 {
                    n1354 = Bundle(22, 0) -> (w1758:cluster{i32, i32})  [unwired: 1 out]
                    n1355 = property class="Tbl (严格)"(reference=w1759, "Index Values"=w1758) -> ()  [unwired: 1 in, 2 out]
                  }
                  frame #1 {
                    n1356 = for {
                      N: 40 -> [_]
                      tunnel: w1761 -> [w1768]
                      i -> [w1763]
                      n1357 = Compound Arithmetic op=ADD(0 ("值"), w1763) -> (w1765:i32)
                      n1358 = Bundle(w1765, 0) -> (w1767:cluster{i32, i32})  [unwired: 1 out]
                      n1359 = property class="Tbl (严格)"(reference=w1768, "Active Cell"=w1767, "Cell BG Color"=u32 16448250) -> ()  [unwired: 1 in, 2 out]
                    }
                  }
                  frame #2 {
                    n1360 = for {
                      N: 5 -> [_]
                      tunnel: w1770 -> [w1777]
                      i -> [w1773]
                      n1361 = Add(x=22, y=w1773) -> (x+y=w1772:i32)
                      n1362 = Bundle(w1772, 0) -> (w1776:cluster{i32, i32})  [unwired: 1 out]
                      n1363 = property class="Tbl (严格)"(reference=w1777, "Active Cell"=w1776, "Cell BG Color"=u32 6618880) -> ()  [unwired: 1 in, 2 out]
                    }
                  }
                }
                n1364 = Select(t=0, s=w1744, f=1) -> (s? t:f=w1743:i32)
                n1365 = property on="项目信息 2" class="Tbl (严格)"("Disabled"=w1743) -> ()  [unwired: 2 in, 2 out]
                n1366 = property on="加热控制参数" class="Clust (严格)"("Disabled"=2) -> ()  [unwired: 2 in, 2 out]
                n1367 = global read "功能码全局.vi" "15"() -> (w1750:bool[])
                n1368 = Index Array(array=w1750, index #1=1 ("索引"), index #2=5 ("索引")) -> (element #1=w1748:bool, element #2=w1747:bool)
                n1369 = Not(x=w1741) -> (.not. x?=w1754:bool)
              }
              frame "保险位置" {
                w1778 = FALSE ("1 6")
                n1370 = control-ref of="项目信息 2"() -> (w1789:refnum<vi>)
                n1371 = stacked-sequence {
                  tunnel: w1789 -> [w1796 w1798 w1807]
                  frame #0 {
                    n1372 = Bundle(0, 0) -> (w1795:cluster{i32, i32})  [unwired: 1 out]
                    n1373 = property class="Tbl (严格)"(reference=w1796, "Index Values"=w1795) -> ()  [unwired: 1 in, 2 out]
                  }
                  frame #1 {
                    n1374 = for {
                      N: 40 -> [_]
                      tunnel: w1798 -> [w1805]
                      i -> [w1801]
                      n1375 = Add(x=2, y=w1801) -> (x+y=w1800:i32)
                      n1376 = Bundle(w1800, 0) -> (w1804:cluster{i32, i32})  [unwired: 1 out]
                      n1377 = property class="Tbl (严格)"(reference=w1805, "Active Cell"=w1804, "Cell BG Color"=u32 16448250) -> ()  [unwired: 1 in, 2 out]
                    }
                  }
                  frame #2 {
                    n1378 = for {
                      N: 20 -> [_]
                      tunnel: w1807 -> [w1814]
                      i -> [w1810]
                      n1379 = Add(x=2, y=w1810) -> (x+y=w1809:i32)
                      n1380 = Bundle(w1809, 0) -> (w1813:cluster{i32, i32})  [unwired: 1 out]
                      n1381 = property class="Tbl (严格)"(reference=w1814, "Active Cell"=w1813, "Cell BG Color"=u32 6618880) -> ()  [unwired: 1 in, 2 out]
                    }
                  }
                }
                n1382 = property on="从板号" class="DigNum (严格)"("NumText.BGColor"=u32 16777215) -> ()  [unwired: 2 in, 2 out]
                n1383 = Select(t=0, s=w1781, f=1) -> (s? t:f=w1780:i32)
                n1384 = property on="项目信息 2" class="Tbl (严格)"("Disabled"=w1780) -> ()  [unwired: 2 in, 2 out]
                n1385 = property on="加热控制参数" class="Clust (严格)"("Disabled"=2) -> ()  [unwired: 2 in, 2 out]
                n1386 = global read "功能码全局.vi" "15"() -> (w1787:bool[])
                n1387 = Index Array(array=w1787, index #1=2 ("索引"), index #2=6 ("索引")) -> (element #1=w1785:bool, element #2=w1784:bool)
                n1388 = Not(x=w1778) -> (.not. x?=w1791:bool)
              }
              frame "温度个数" {
                w1815 = FALSE ("1 6")
                n1389 = control-ref of="项目信息 2"() -> (w1826:refnum<vi>)
                n1390 = stacked-sequence {
                  tunnel: w1826 -> [w1833 w1834 w1844]
                  frame #0 {
                    n1391 = Bundle(0, 0) -> (w1832:cluster{i32, i32})  [unwired: 1 out]
                    n1392 = property class="Tbl (严格)"(reference=w1833, "Index Values"=w1832) -> ()  [unwired: 1 in, 2 out]
                  }
                  frame #1 {
                    n1393 = for {
                      N: 40 -> [_]
                      tunnel: w1834 -> [w1842]
                      i -> [w1837]
                      n1394 = Compound Arithmetic op=ADD(0 ("值"), w1837) -> (w1839:i32)
                      n1395 = Bundle(w1839, 0) -> (w1841:cluster{i32, i32})  [unwired: 1 out]
                      n1396 = property class="Tbl (严格)"(reference=w1842, "Active Cell"=w1841, "Cell BG Color"=u32 16448250) -> ()  [unwired: 1 in, 2 out]
                    }
                  }
                  frame #2 {
                    n1397 = for {
                      N: 1 -> [_]
                      tunnel: w1844 -> [w1851]
                      i -> [w1847]
                      n1398 = Add(x=1, y=w1847) -> (x+y=w1846:i32)
                      n1399 = Bundle(w1846, 0) -> (w1850:cluster{i32, i32})  [unwired: 1 out]
                      n1400 = property class="Tbl (严格)"(reference=w1851, "Active Cell"=w1850, "Cell BG Color"=u32 6618880) -> ()  [unwired: 1 in, 2 out]
                    }
                  }
                }
                n1401 = Select(t=0, s=w1818, f=1) -> (s? t:f=w1817:i32)
                n1402 = property on="项目信息 2" class="Tbl (严格)"("Disabled"=w1817) -> ()  [unwired: 2 in, 2 out]
                n1403 = property on="加热控制参数" class="Clust (严格)"("Disabled"=2) -> ()  [unwired: 2 in, 2 out]
                n1404 = property on="从板号" class="DigNum (严格)"("NumText.BGColor"=u32 16777215) -> ()  [unwired: 2 in, 2 out]
                n1405 = global read "功能码全局.vi" "15"() -> (w1824:bool[])
                n1406 = Index Array(array=w1824, index #1=3 ("索引"), index #2=7 ("索引")) -> (element #1=w1822:bool, element #2=w1821:bool)
                n1407 = Not(x=w1815) -> (.not. x?=w1828:bool)
              }
              frame "SOC过低", "电压不均衡", "电压过低", "电压过高", "温度不均衡", "温度过低", "温度过高", "一级故障阀值" {
                w1852 = FALSE ("1 6")
                n1408 = property on="从板号" class="DigNum (严格)"("NumText.BGColor"=u32 16777215) -> ()  [unwired: 2 in, 2 out]
                n1409 = Select(t=0, s=w1854, f=1) -> (s? t:f=w1855:i32)
                n1410 = property on="一级故障 6" class="Clust (严格)"("DisabledEnum"=w1855) -> ()  [unwired: 2 in, 2 out]
                n1411 = global read "功能码全局.vi" "18"() -> (w1861:bool[])
                n1412 = Index Array(array=w1861, index #1=2 ("索引"), index #2=5 ("索引")) -> (element #1=w1859:bool, element #2=w1858:bool)
                n1413 = Not(x=w1852) -> (.not. x?=w1863:bool)
              }
              frame "SOC过低(2)", "电压不均衡(2)", "电压过低(2)", "电压过高(2)", "二级故障阀值", "温度不均衡(2)", "温度过低(2)", "温度过高(2)" {
                w1865 = FALSE ("1 6")
                n1414 = property on="从板号" class="DigNum (严格)"("NumText.BGColor"=u32 16777215) -> ()  [unwired: 2 in, 2 out]
                n1415 = Select(t=0, s=w1868, f=1) -> (s? t:f=w1867:i32)
                n1416 = property on="一级故障 7" class="Clust (严格)"("DisabledEnum"=w1867) -> ()  [unwired: 2 in, 2 out]
                n1417 = global read "功能码全局.vi" "18"() -> (w1874:bool[])
                n1418 = Index Array(array=w1874, index #1=3 ("索引"), index #2=6 ("索引")) -> (element #1=w1872:bool, element #2=w1871:bool)
                n1419 = Not(x=w1865) -> (.not. x?=w1876:bool)
              }
              frame "SOC过低(3)", "电压不均衡(3)", "电压过低(3)", "电压过高(3)", "三级故障阀值", "温度不均衡(3)", "温度过低(3)", "温度过高(3)" {
                w1878 = FALSE ("1 6")
                n1420 = property on="从板号" class="DigNum (严格)"("NumText.BGColor"=u32 16777215) -> ()  [unwired: 2 in, 2 out]
                n1421 = Select(t=0, s=w1881, f=1) -> (s? t:f=w1880:i32)
                n1422 = property on="一级故障 8" class="Clust (严格)"("DisabledEnum"=w1880) -> ()  [unwired: 2 in, 2 out]
                n1423 = global read "功能码全局.vi" "18"() -> (w1887:bool[])
                n1424 = Index Array(array=w1887, index #1=4 ("索引"), index #2=7 ("索引")) -> (element #1=w1885:bool, element #2=w1884:bool)
                n1425 = Not(x=w1878) -> (.not. x?=w1889:bool)
              }
              frame "快换参数" {
                w1891 = FALSE ("1 6")
                n1426 = Select(t=0, s=w1912, f=1) -> (s? t:f=w1911:i32)
                n1427 = property on="电池组信息" class="Clust (严格)"("Disabled"=w1911) -> ()  [unwired: 2 in, 2 out]
                n1428 = property on="从板号" class="DigNum (严格)"("NumText.BGColor"=u32 16777215) -> ()  [unwired: 2 in, 2 out]
                n1429 = global read "功能码全局.vi" "24"() -> (w1908:bool[])
                n1430 = global read "功能码全局.vi" "23"() -> (w1909:bool[])
                n1431 = Index Array(array=w1908) -> (element #3=w1898:bool, element #4=w1897:bool, element #5=w1896:bool, element #6=w1895:bool, element #7=w1894:bool, element #8=w1893:bool)  [unwired: 8 in, 2 out]
                n1432 = Index Array(array=w1909) -> (element #3=w1907:bool, element #4=w1906:bool, element #5=w1905:bool, element #6=w1904:bool, element #7=w1903:bool, element #8=w1902:bool)  [unwired: 8 in, 2 out]
